vi "InitializeObstacleArrays.vi"() -> (2 "Obstacle Points of Interest":T3[](array[typedef]) {"North" format="%#_10f"; "East" format="%#_8f"}, 3 "Obstacle Arrays Cluster":T1 {"Readable Obstacles"."Obstacle Array"."North" format="%#_10f"; "Readable Obstacles"."Obstacle Array"."East" format="%#_8f"})   [LabVIEW 2013]
doc: "This initializes the arrays that are used for obstacle tracking and packs them into a cluster. It also initializes an empty UTM array for wiping points of interest in the future.\n\nEric Schneider, August 2014"
uses:
  cRIO_Code/Data/TypeDefs/UTM Location.ctl
  TypeDef/obstacle_arrays.ctl
  cRIO_Code/Logic/Classes/Obstacle/Obstacle.lvclass
  cRIO_Code/Data/TypeDefs/ObstacleDescription.ctl
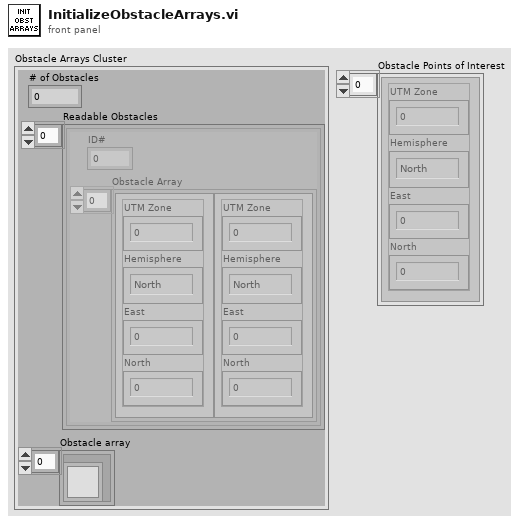
[diagram p1: front panel]
types:
  T1 = typedef "obstacle_arrays.ctl" = cluster{"# of Obstacles":i32, "Obstacle array":refnum<class "Obstacle.lvclass">[], "Readable Obstacles":T2[]}
  T2 = typedef "ObstacleDescription.ctl" = cluster{"ID#":i32, "Obstacle Array":T3[]}
  T3 = typedef "UTM Location.ctl" = cluster{"UTM Zone":dbl, "Hemisphere":enum16{"North", "South"}, "East":dbl, "North":dbl}
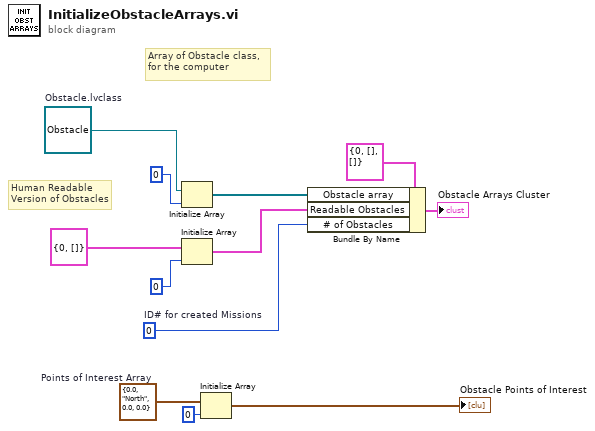
[diagram p0: block diagram]
diagram:
  w4 = refnum<class "Obstacle.lvclass"> refnum  # Obstacle.lvclass
  w8 = T3 {"UTM Zone"=0.0, "Hemisphere"=enum."North", "East"=0.0, "North"=0.0}  # Points of Interest Array
  w10 = 0  # ID# for created Missions
  # "Array of Obstacle class, for the computer"
  # "Human Readable Version of Obstacles"
  n1 = Initialize Array "Initialize Array"(w4, 0 ("dimension size")) -> (w9:refnum<class "Obstacle.lvclass">[])
  n2 = Initialize Array "Initialize Array"(T2 {"ID#"=0, "Obstacle Array"=[]} ("Human Readable Obstacle Cluster"), 0 ("dimension size")) -> (w2:T2[])
  n3 = Initialize Array(w8, 0 ("dimension size")) -> (→"Obstacle Points of Interest":T3[])
  n4 = Bundle By Name(cluster=T1 {"# of Obstacles"=0, "Obstacle array"=[], "Readable Obstacles"=[]} ("Obstacle Arrays Cluster"), "Obstacle array"=w9, "Readable Obstacles"=w2, "# of Obstacles"=w10) -> (→"Obstacle Arrays Cluster":T1)
